vi "SetProperty.vi"(8 "error in (no error)":errorcluster, 9 "Value of Property":string, 10 "Property":string, 11 "Thing Info In":T2) -> (0 "error out":errorcluster, 3 "Thing Info Out":T2)   [LabVIEW 2015]
uses:
  <vilib>/httpClient/ClientHandle.ctl
  <vilib>/httpClient/PUTBuffer.vi
  <vilib>/httpClient/LabVIEWHTTPClient.lvlib
panel:
  out "body":string
  out "Final url":string
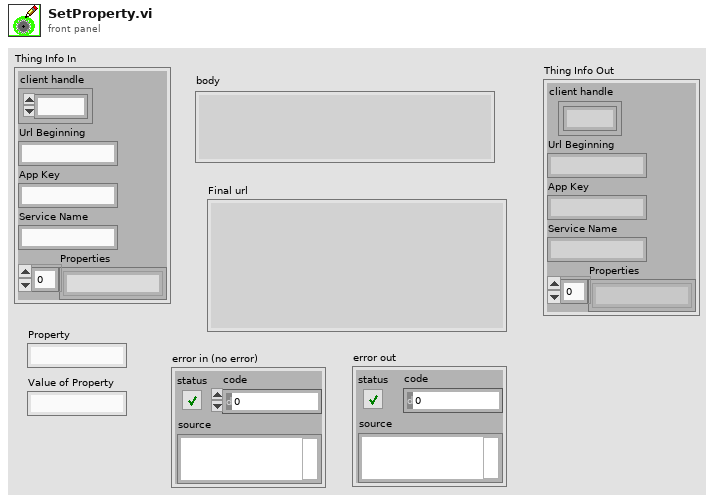
[diagram p1: front panel]
types:
  T1 = typedef "LabVIEWHTTPClient.lvlib/ClientHandle.ctl" = refnum<k1>
  T2 = cluster{"client handle":T1, "Url Beginning":string, "App Key":string, "Service Name":string, "Properties":string[]}
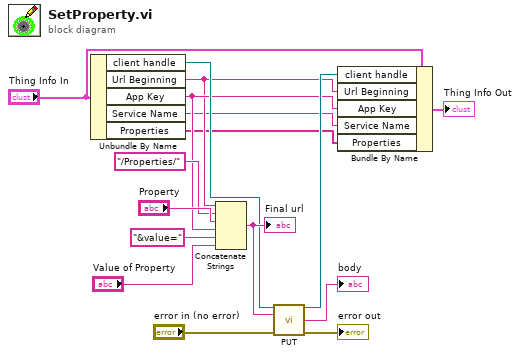
[diagram p0: block diagram]
diagram:
  n1 = Unbundle By Name("Thing Info In") -> ("client handle"=w8:T1, "Url Beginning"=w3:string, "App Key"=w4:string, "Service Name"=w2:string, "Properties"=w1:string[])
  n2 = Concatenate Strings(w3, "/Properties/" ("string"), "Property", w4, "&value=" ("string"), "Value of Property") -> (w14:string)
  "Final url" <- w14
  n3 = call-poly <vilib>:"PUT.vi"("client handle"=w8, "url"=w14, "error in (no error)"="error in (no error)") -> ("client handle out"=w7:T1, "body"=→"body":string, "error out"=→"error out":errorcluster)  [unwired: 9 in, 1 out]
  n4 = Bundle By Name(cluster="Thing Info In", "client handle"=w7, "Url Beginning"=w3, "App Key"=w4, "Service Name"=w2, "Properties"=w1) -> (→"Thing Info Out":T2)
